vi "Actor Core.vi"(8 "error in":errorcluster, 11 "VolatusCore in":refnum<class "VolatusCore.lvclass">) -> (0 "error out":errorcluster, 3 "Actor out":refnum<class "Actor.lvclass">)   [LabVIEW 2020, in "Volatus.lvlib" / "VolatusCore.lvclass"]
doc: "(<B>Filename</B>: Actor Framework.lvlib:Actor.lvclass:Actor Core.vi)\n\nReceives messages to the actor, reacts to them, and initiates any error handling that may shut the actor down.\n\nDescendant classes may override this VI to append parallel tasks for the actor to complete while it handles messages. Overrides use the Call Parent Class Method node."
uses:
  VolatusCore.lvclass
  <vilib>/ActorFramework/Actor/Actor.lvclass
  C:/Program Files (x86)/National Instruments/LabVIEW 2020/vi.lib/ActorFramework/Actor/Actor.lvclass
  C:/dev/lv20CE/relink/lv-volatus/Volatus/VolatusCore/VolatusCore.lvclass
  C:/dev/lv20CE/relink/lv-volatus/Volatus/APIRegistrationHandler/APIRegistrationHandler.lvclass
  C:/dev/lv20CE/relink/lv-volatus/Volatus/TaskStateHandler/TaskStateHandler.lvclass
  C:/dev/lv20CE/relink/lv-volatus/Volatus/VectoMessageHandler/VectoMessageHandler.lvclass
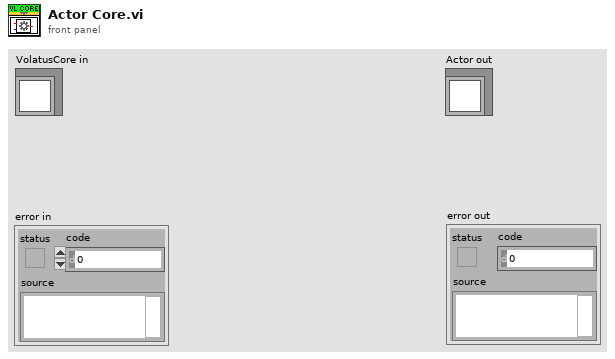
[diagram p1: front panel]
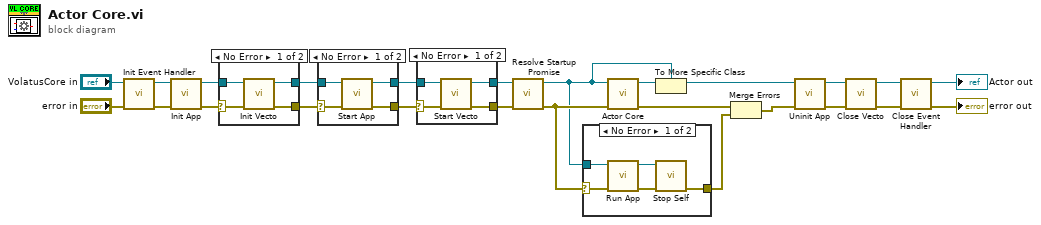
[diagram p0: block diagram]
diagram:
  n1 = call "Init Event Handler.vi"("error in (no error)"="error in", "VolatusCore in"="VolatusCore in") -> ("error out"=w6:errorcluster, "VolatusCore out"=w4:refnum<class "VolatusCore.lvclass">)  [unwired: 8 in]
  n2 = call "Init App.vi"("error in (no error)"=w6, "VolatusCore in"=w4) -> ("error out"=w23:errorcluster, "VolatusCore out"=w21:refnum<class "VolatusCore.lvclass">)  [unwired: 8 in]
  n3 = case shown="No Error" w23 {
    selector: w23 -> [w29 w30]
    tunnel: [w28 w30] -> w22
    tunnel: w21 -> [w27 w31]
    tunnel: [w26 w31] -> w19
    frame No Error {
      n4 = call "Init Vecto.vi"("error in (no error)"=w29, "VolatusCore in"=w27) -> ("error out"=w28:errorcluster, "VolatusCore out"=w26:refnum<class "VolatusCore.lvclass">)  [unwired: 8 in]
    }
    frame Error {
    }
  }
  n5 = case shown="No Error" w22 {
    selector: w22 -> [w35 w36]
    tunnel: [w34 w36] -> w20
    tunnel: w19 -> [w33 w37]
    tunnel: [w32 w37] -> w17
    frame No Error {
      n6 = call "Start App.vi"("error in (no error)"=w35, "VolatusCore in"=w33) -> ("error out"=w34:errorcluster, "VolatusCore out"=w32:refnum<class "VolatusCore.lvclass">)  [unwired: 8 in]
    }
    frame Error {
    }
  }
  n7 = case shown="No Error" w20 {
    selector: w20 -> [w41 w42]
    tunnel: [w40 w42] -> w18
    tunnel: w17 -> [w39 w43]
    tunnel: [w38 w43] -> w16
    frame No Error {
      n8 = call "Start Vecto.vi"("error in (no error)"=w41, "VolatusCore in"=w39) -> ("error out"=w40:errorcluster, "VolatusCore out"=w38:refnum<class "VolatusCore.lvclass">)  [unwired: 8 in]
    }
    frame Error {
    }
  }
  n9 = call "Resolve Startup Promise.vi"("error in (no error)"=w18, "VolatusCore in"=w16) -> ("error out"=w12:errorcluster, "VolatusCore out"=w11:refnum<class "VolatusCore.lvclass">)  [unwired: 8 in]
  n10 = case shown="No Error" w12 {
    selector: w12 -> [w47 _]
    tunnel: w11 -> [w48 _]
    tunnel: [w44 _] -> w9
    frame No Error {
      n11 = call "Run App.vi"("error in (no error)"=w47, "VolatusCore in"=w48) -> ("error out"=w45:errorcluster, "VolatusCore out"=w46:refnum<class "VolatusCore.lvclass">)  [unwired: 8 in]
      n12 = call "Stop Self.vi"("error in (no error)"=w45, "VolatusCore in"=w46) -> ("error out"=w44:errorcluster)  [unwired: 8 in, 1 out]
    }
    frame Error {
    }
  }
  n13 = call-parent "Actor Core.vi"("error in"=w12, "Actor in"=w11) -> ("error out"=w24:errorcluster, "Actor out"=w15:refnum<class "Actor.lvclass">)  [unwired: 8 in]
  n14 = To More Specific Class(target class=w11, reference=w15) -> (specific class reference=w13:refnum<class "VolatusCore.lvclass">)  [unwired: 1 in, 1 out]
  n15 = Merge Errors(w24, w9) -> (w10:errorcluster)
  n16 = call "Uninit App.vi"("error in (no error)"=w10, "VolatusCore in"=w13) -> ("error out"=w14:errorcluster, "VolatusCore out"=w7:refnum<class "VolatusCore.lvclass">)  [unwired: 8 in]
  n17 = call "Close Vecto.vi"("error in (no error)"=w14, "VolatusCore in"=w7) -> ("error out"=w8:errorcluster, "VolatusCore out"=w2:refnum<class "VolatusCore.lvclass">)  [unwired: 8 in]
  n18 = call "Close Event Handler.vi"("error in (no error)"=w8, "VolatusCore in"=w2) -> ("error out"=→"error out":errorcluster, "VolatusCore out"=→"Actor out":refnum<class "VolatusCore.lvclass">)  [unwired: 8 in]
